vi "S2C_ExeScriptFormatResult.vi"(8 "Error In":errorcluster, 11 "Q-Ref":refnum<queue>) -> (0 "Error Out":errorcluster)   [LabVIEW 2015]
doc: "Resets relevant controls at the termination of execution, and displays the results banner."
uses:
  Controls/S2C_ExePause.ctl
  Globals/S2C_Globals.vi
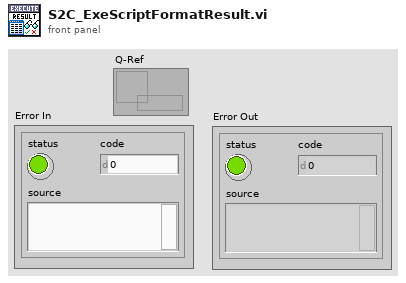
[diagram p1: front panel]
types:
  T1 = typedef "S2C_ExePause.ctl" = bool
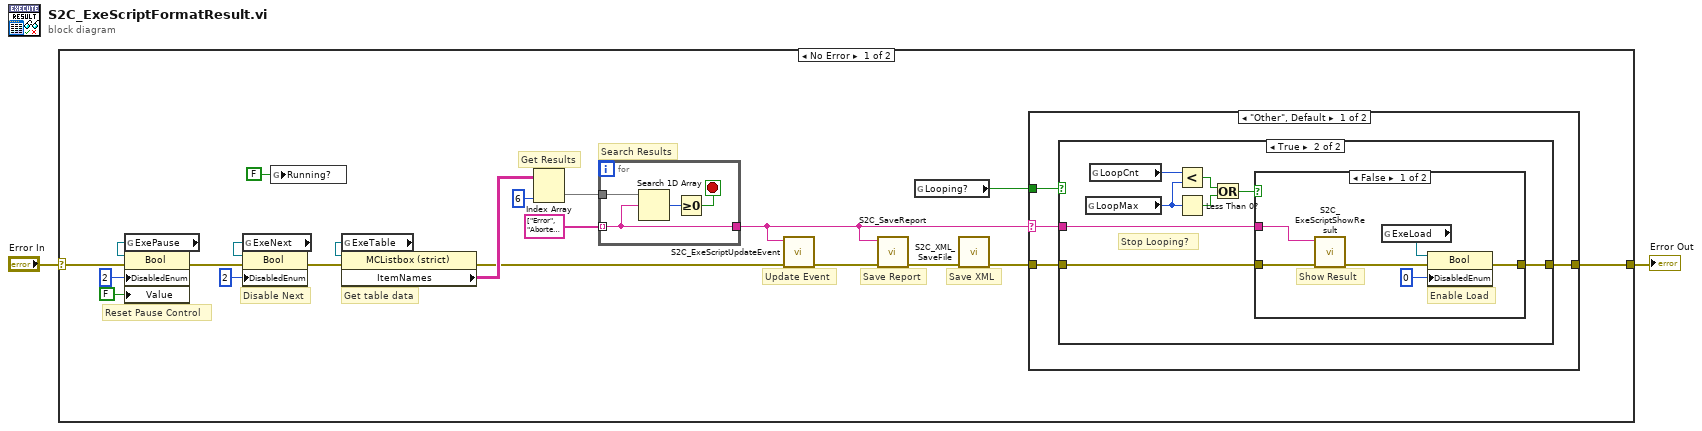
[diagram p0: block diagram]
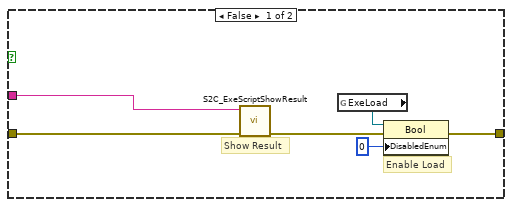
[diagram p2: hidden frame]
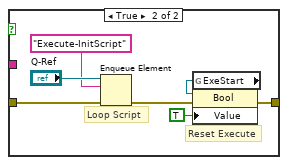
[diagram p3: hidden frame]
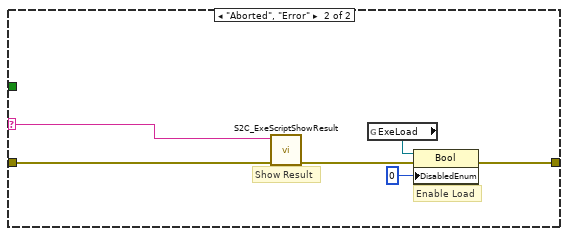
[diagram p4: hidden frame]
diagram:
  n1 = case shown="No Error" "Error In" {
    selector: "Error In" -> [w12 w65]
    tunnel: [w23 w65] -> w1
    frame No Error {
      # "Update Event"
      # "Save XML"
      # "Save Report"
      # "Get Results"
      # "Reset Pause Control"
      # "Disable Next"
      # "Search Results"
      # "Get table data"
      n2 = global read "S2C_Globals.vi" "ExePause"() -> (w15:refnum<vi>)
      n3 = property on="Property Node" class="Bool"(reference=w15, error in=w12, "DisabledEnum"=u8 2, "Value"=T1 FALSE) -> (error out=w13:errorcluster)  [unwired: 1 out]
      n4 = global read "S2C_Globals.vi" "ExeNext"() -> (w18:refnum<vi>)
      n5 = property on="Property Node" class="Bool"(reference=w18, error in=w13, "DisabledEnum"=u8 2) -> (error out=w11:errorcluster)  [unwired: 1 out]
      n6 = global write "S2C_Globals.vi" "Running?"(FALSE ("Running?")) -> ()
      n7 = global read "S2C_Globals.vi" "ExeTable"() -> (w22:refnum<vi>)
      n8 = property class="MCListbox (strict)"(reference=w22, error in=w11) -> (error out=w5:errorcluster, "ItemNames"=w21:string[][])  [unwired: 1 out]
      n9 = Index Array(array=w21, index (col)=6 ("disabled index (col)")) -> (element=w19:string[])  [unwired: 1 in]
      n10 = for {
        tunnel: w19 -> [w64]
        tunnel: string[] ["Error", "Aborted", "Failed", "Passed", "Logged", "No Record"] -> [w61] mode=indexing
        tunnel: [w61] -> w3
        stop <- w62 stop-if-true
        n11 = Search 1D Array(1D array=w64, element=w61) -> (index of element=w63:i32)  [unwired: 1 in]
        n12 = Greater Or Equal To 0?(x=w63) -> (x >= 0?=w62:bool)
      }
      n13 = call "S2C_ExeScriptUpdateEvent.vi"("Error In"=w5, "Result"=w3) -> ("Error Out"=w4:errorcluster)  [unwired: 9 in]
      n14 = call "S2C_SaveReport.vi"("Error In"=w4, "Result"=w3) -> ("Error Out"=w8:errorcluster)  [unwired: 9 in]
      n15 = global read "S2C_Globals.vi" "Looping?"() -> (w10:bool)
      n16 = call "S2C_XML_SaveFile.vi"("Error In"=w8) -> ("Error Out"=w7:errorcluster)  [unwired: 10 in]
      n17 = case shown="\"Other\", Default" w3 {
        selector: w3 -> [w24 w59]
        tunnel: [w27 w55] -> w23
        tunnel: w7 -> [w26 w60]
        tunnel: w10 -> [w25 _]
        frame "Other", Default {
          n18 = case shown="True" w25 {
            tunnel: [w28 w40] -> w27
            tunnel: w26 -> [w33 w41]
            tunnel: w24 -> [w32 w38]
            frame False {
              # "Enable Load"
              # "Show Result"
              n19 = call "S2C_ExeScriptShowResult.vi"("Error In"=w33, "Result In"=w32) -> ("Error Out"=w29:errorcluster)  [unwired: 9 in]
              n20 = global read "S2C_Globals.vi" "ExeLoad"() -> (w30:refnum<vi>)
              n21 = property class="Bool"(reference=w30, error in=w29, "DisabledEnum"=u8 0) -> (error out=w28:errorcluster)  [unwired: 1 out]
            }
            frame True {
              # "Stop Looping?"
              n22 = global read "S2C_Globals.vi" "LoopMax"() -> (w37:i32)
              n23 = global read "S2C_Globals.vi" "LoopCnt"() -> (w39:i32)
              n24 = Less?(x=w39, y=w37) -> (x < y?=w36:bool)
              n25 = Less Than 0?(x=w37) -> (x < 0?=w35:bool)
              n26 = Or(x=w36, y=w35) -> (x .or. y?=w34:bool)
              n27 = case shown="False" w34 {
                tunnel: w41 -> [w47 w54]
                tunnel: [w42 w48] -> w40
                tunnel: w38 -> [w46 _]
                frame False {
                  # "Enable Load"
                  # "Show Result"
                  n28 = call "S2C_ExeScriptShowResult.vi"("Error In"=w47, "Result In"=w46) -> ("Error Out"=w43:errorcluster)  [unwired: 9 in]
                  n29 = global read "S2C_Globals.vi" "ExeLoad"() -> (w44:refnum<vi>)
                  n30 = property class="Bool"(reference=w44, error in=w43, "DisabledEnum"=u8 0) -> (error out=w42:errorcluster)  [unwired: 1 out]
                }
                frame True {
                  # "Loop Script"
                  # "Reset Execute"
                  n31 = Enqueue Element(queue="Q-Ref", element="Execute-InitScript", error in (no error)=w54) -> (error out=w49:errorcluster)  [unwired: 1 in, 2 out]
                  n32 = global read "S2C_Globals.vi" "ExeStart"() -> (w52:refnum<vi>)
                  n33 = property on="Property Node" class="Bool"(reference=w52, error in=w49, "Value"=TRUE) -> (error out=w48:errorcluster)  [unwired: 1 out]
                }
              }
            }
          }
        }
        frame "Aborted", "Error" {
          # "Enable Load"
          # "Show Result"
          n34 = call "S2C_ExeScriptShowResult.vi"("Error In"=w60, "Result In"=w59) -> ("Error Out"=w56:errorcluster)  [unwired: 9 in]
          n35 = global read "S2C_Globals.vi" "ExeLoad"() -> (w57:refnum<vi>)
          n36 = property class="Bool"(reference=w57, error in=w56, "DisabledEnum"=u8 0) -> (error out=w55:errorcluster)  [unwired: 1 out]
        }
      }
    }
    frame Error {
    }
  }
  "Error Out" <- w1
